vi "一体站流程自动启动.vi"(11 "参数":T1={"CODCr"={"启动测量模式"={"测量模式"=enum."水样测量"}, "确定按钮"=TRUE}, "参数启用"={"多参数"=FALSE, "CODMn"=FALSE, "总磷总氮"=FALSE, "氨氮"=FALSE, "CODcr"=FALSE}}) -> ()   [LabVIEW 2016, in "PLC.lvlib"]
uses:
  PLC.lvlib
  API/CodCr/CodCr.lvlib
panel:
  out "枚举":enum16{"初始化", "采配水启动", "等待", "配水", "排水", "结束"}(ring)
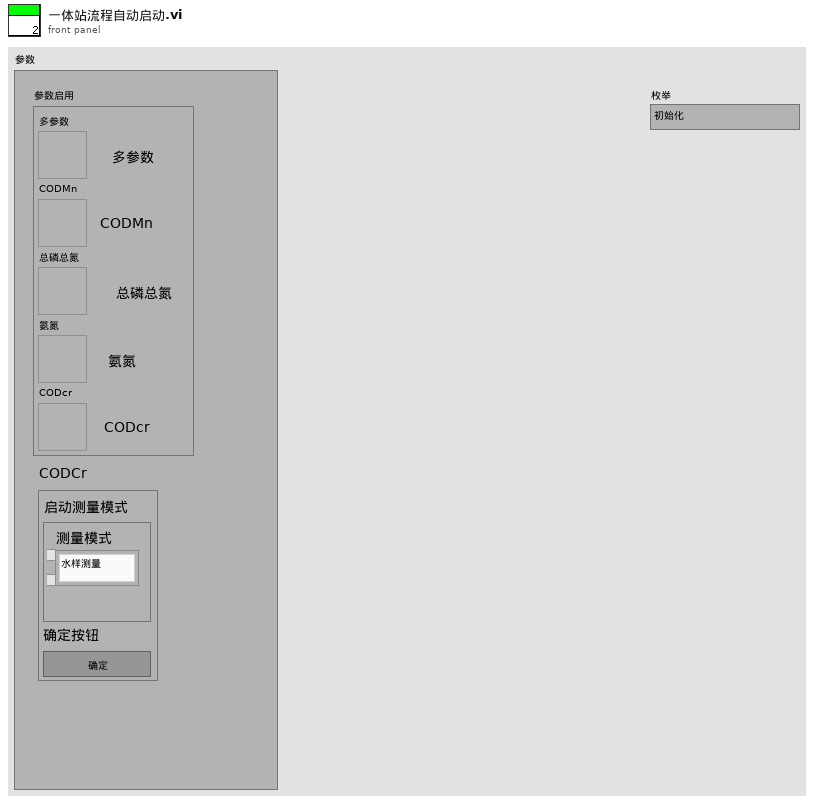
[diagram p1: front panel]
types:
  T1 = cluster{"CODCr":cluster{"启动测量模式":cluster{"测量模式":enum16{"水样测量", "标样核查", "零点核查", "跨度核查", "加标回收", "平行样", "校零", "校标"}}, "确定按钮":bool}, "参数启用":cluster{"多参数":bool, "CODMn":bool, "总磷总氮":bool, "氨氮":bool, "CODcr":bool}}
  T2 = cluster{"命令":string, cluster{"starting address":u16, "holding register value":u16}}
  T3 = cluster{"测量模式":enum16{"水样测量", "标样核查", "零点核查", "跨度核查", "空白测试", "加标回收", "平行样", "校零", "校标"}}
  T4 = cluster{"时间标识":timestamp, "设备":string, "日志信息":string, "流程参数":string}
  T5 = cluster{"时间标识":timestamp, "设备":string, "日志信息":string}
  T6 = enum16{"空闲", "水样测试", "标样核查", "零点核查", "跨度核查", "空白测试", "平行样测试", "加标回收", "空白校准", "标样校准", "初始化（清洗）"}
  T7 = enum16{"待机", "启动氨氮", "氨氮测量中", "启动总磷", "总磷测量中", "结束"}
  T8 = cluster{"站号":u16, "量程切换":enum32{"H", "L", "AUTO"}, "控制命令":enum16{"启动测量", "标样核查", "零点核查", "跨度核查", "空白测试", "平行样测试", "加标回收", "空白校准", "标样校准", "初始化（清洗）", "停止测试", "仪器重启", "校时", "模式设置", "测量间隔设置"}, "模式设置":enum16{"待机", "连续模式", "周期模式", "定点模式", "受控模式", "手动模式"}, "测量间隔":u16}
  T9 = cluster{"测量模式":enum16{"待机", "水样测试", "标样核查", "零点核查", "跨度核查", "空白测试", "平行样测试", "加标回收", "空白校准", "标样校准", "初始化（清洗）"}, "数据标记表":string, "测量时间":dbl}
  T10 = enum16{"待机", "水样测试", "标样核查", "零点核查", "跨度核查", "空白测试", "平行样测试", "加标回收", "空白校准", "标样校准", "初始化（清洗）"}
  T11 = cluster{"R0":i16, "R1":i16, "R2":i16, "R3":i16, "R4":i16, "R5":i16, "R6":i16, "R7":i16, "R8":i16, "R9":i16, "R10":i16, "R11":i16, "R12":i16, "R13":i16, "R14":i16, "R15":i16, "R16":i16, "R17":i16, "R18":i16, "R19":i16, "R20":i16, "R21":i16, "R22":i16, "R23":i16, "R24":i16, "R25":i16}
  T12 = enum32{"Bad", "Idle", "Run top level", "Running"}
  T13 = cluster{"系统时间":timestamp, "工作状态":enum16{"空闲", "水样测试", "标样核查", "零点核查", "跨度核查", "空白测试", "平行样测试", "加标回收", "空白校准", "标样校准", "初始化（清洗）"}, "测量模式":enum16{"待机", "连续模式", "周期模式", "定点模式", "受控模式", "手动模式"}, "告警代码":enum16{"无告警", "缺试剂告警", "缺水样告警", "缺蒸馏水告警", "缺标液告警", "仪表漏液告警", "标定异常告警", "超量程告警", "加热异常", "低试剂预警", "超上限告警", "超下限告警", "仪表内部其他异常", "滴定异常告警", "电极异常告警", "量程切换告警", "参数设置告警", "PH电极电位异常", "电导率电极异常", "浊度光度异常", "溶解氧电极异常", "溶解氧光强异常", "温度异常告警", "PH异常告警", "溶解氧异常告警", "电导率异常告警", "浊度异常告警", "叶绿素异常告警", "藻密度异常告警", "蓝绿藻异常告警", "ORP异常告警", "氨氮异常告警", "清洁刷异常告警", "SD卡异常告警", "蓝牙异常告警", "Wifi异常告警", "流程异常告警"}, "故障代码":enum16{"无故障", "电机故障", "温度故障", "通讯故障", "滴定故障"}, "日志代码":u16, "软件版本":u16, "F0":sgl, "F1":sgl, "F2":sgl, "F3":sgl, "T":sgl, "H":sgl, "id":u16, "flowid":u16, "量程":u16}
  T14 = cluster{"测量模式":enum16{"水样测量", "标样核查", "零点核查", "跨度核查", "加标回收", "平行样", "校零", "校标"}}
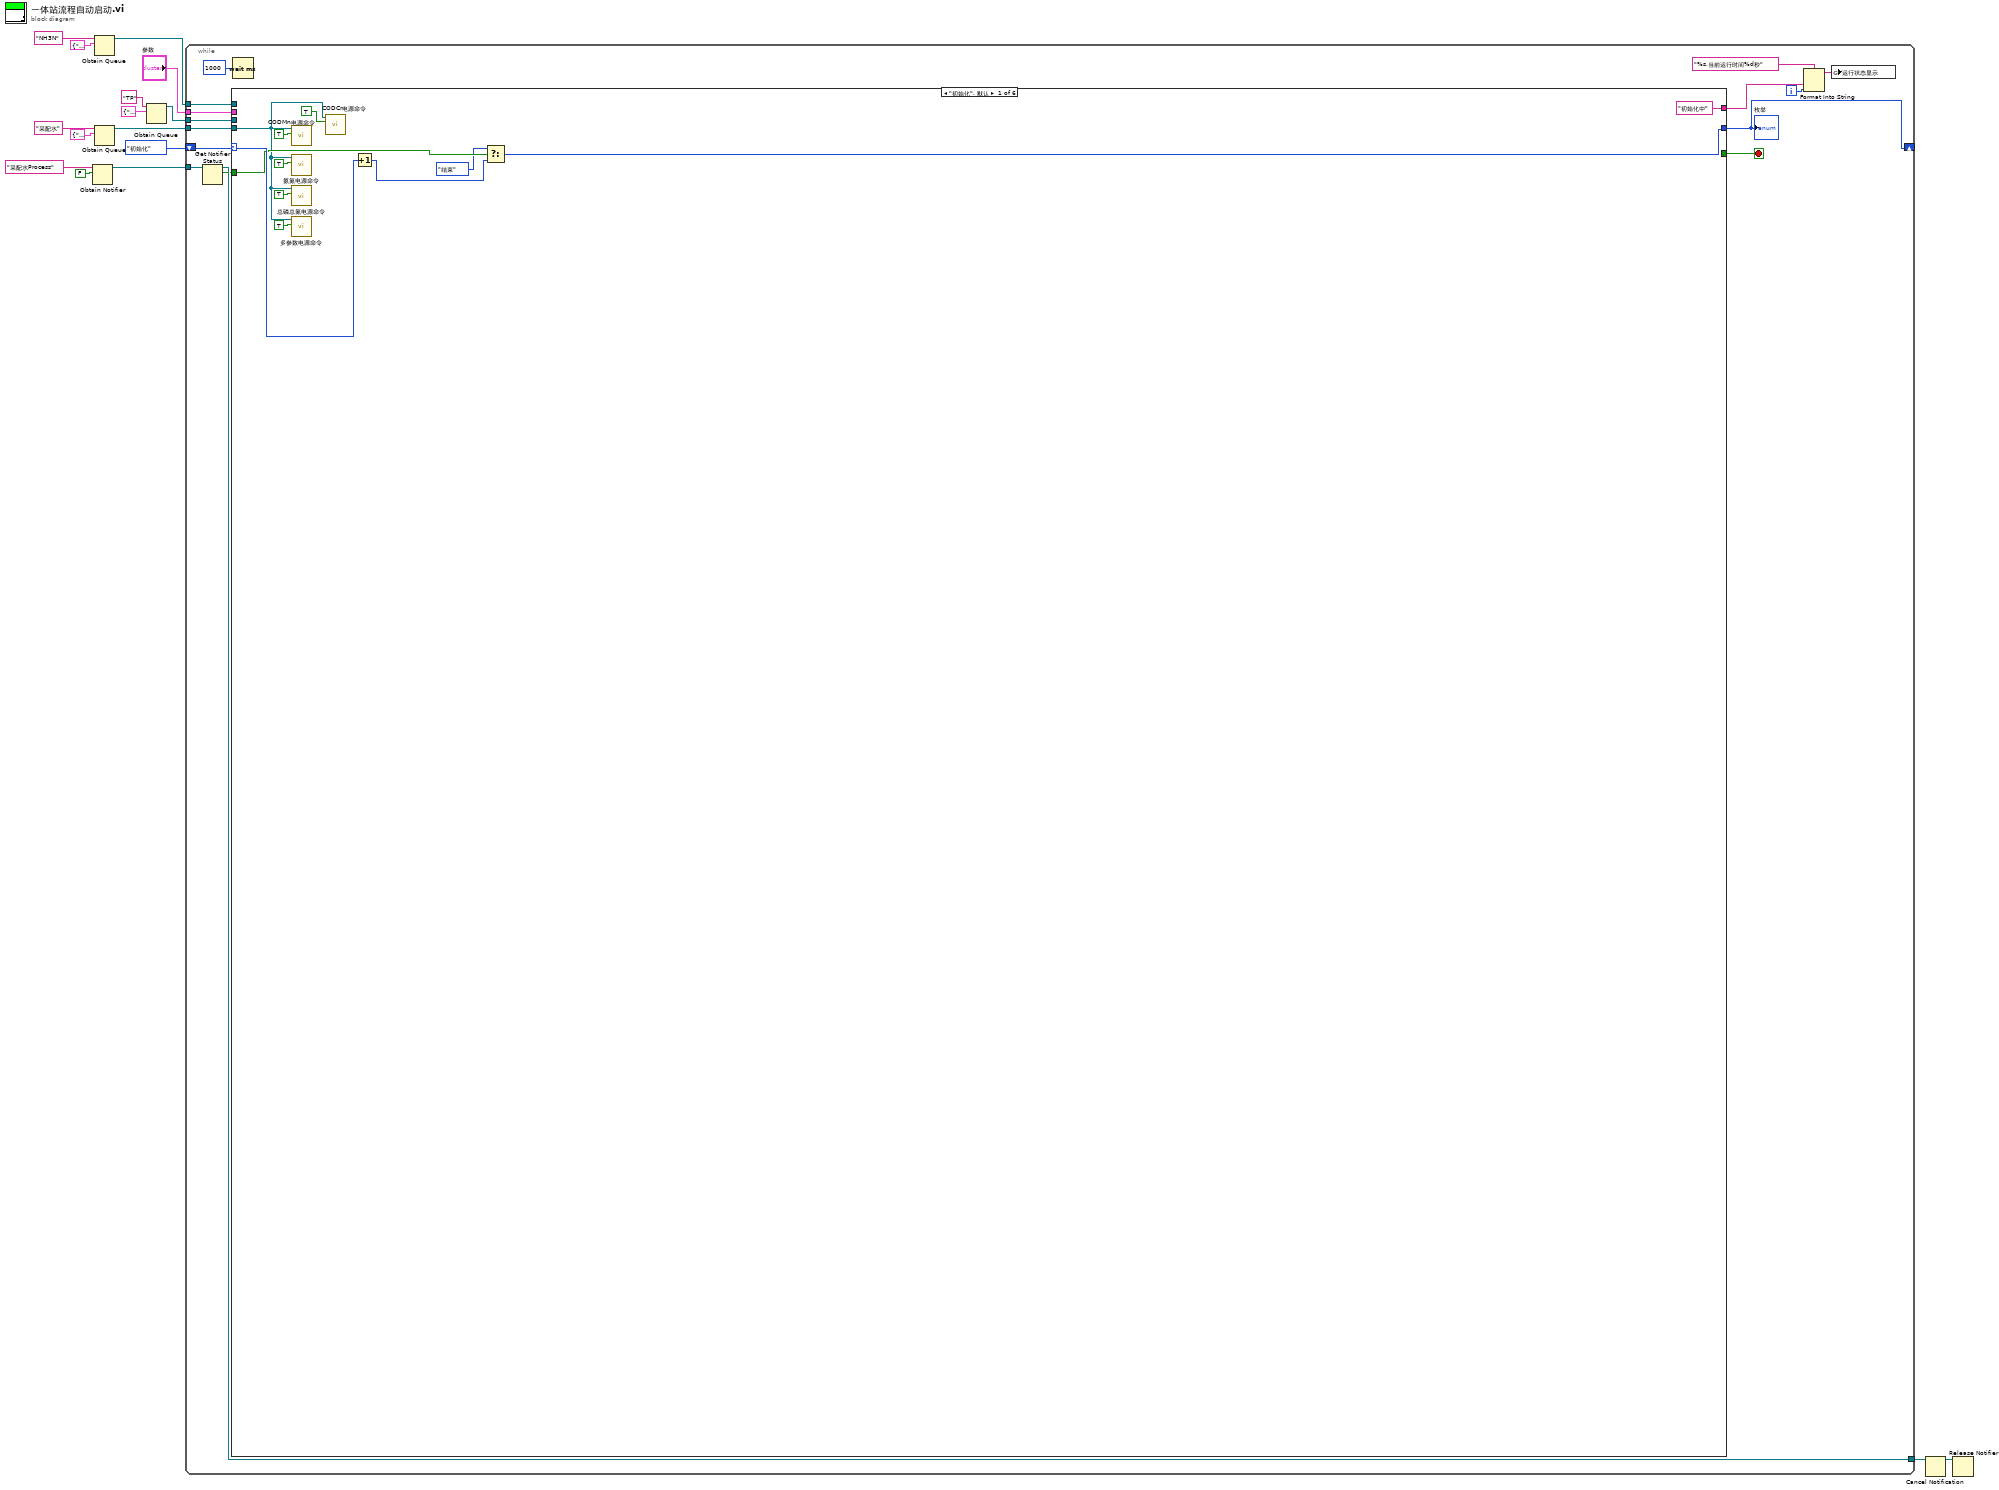
[diagram p0: block diagram]
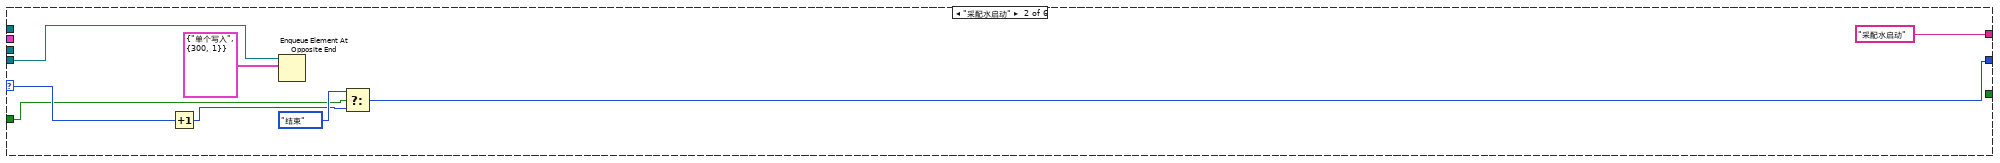
[diagram p2: hidden frame]
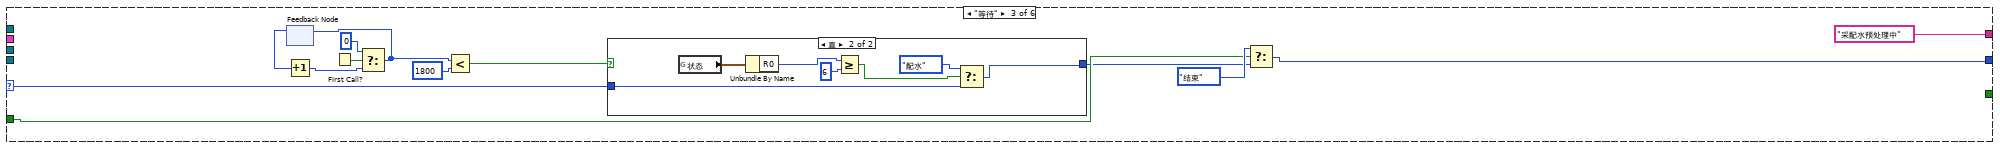
[diagram p3: hidden frame]
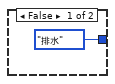
[diagram p4: hidden frame]
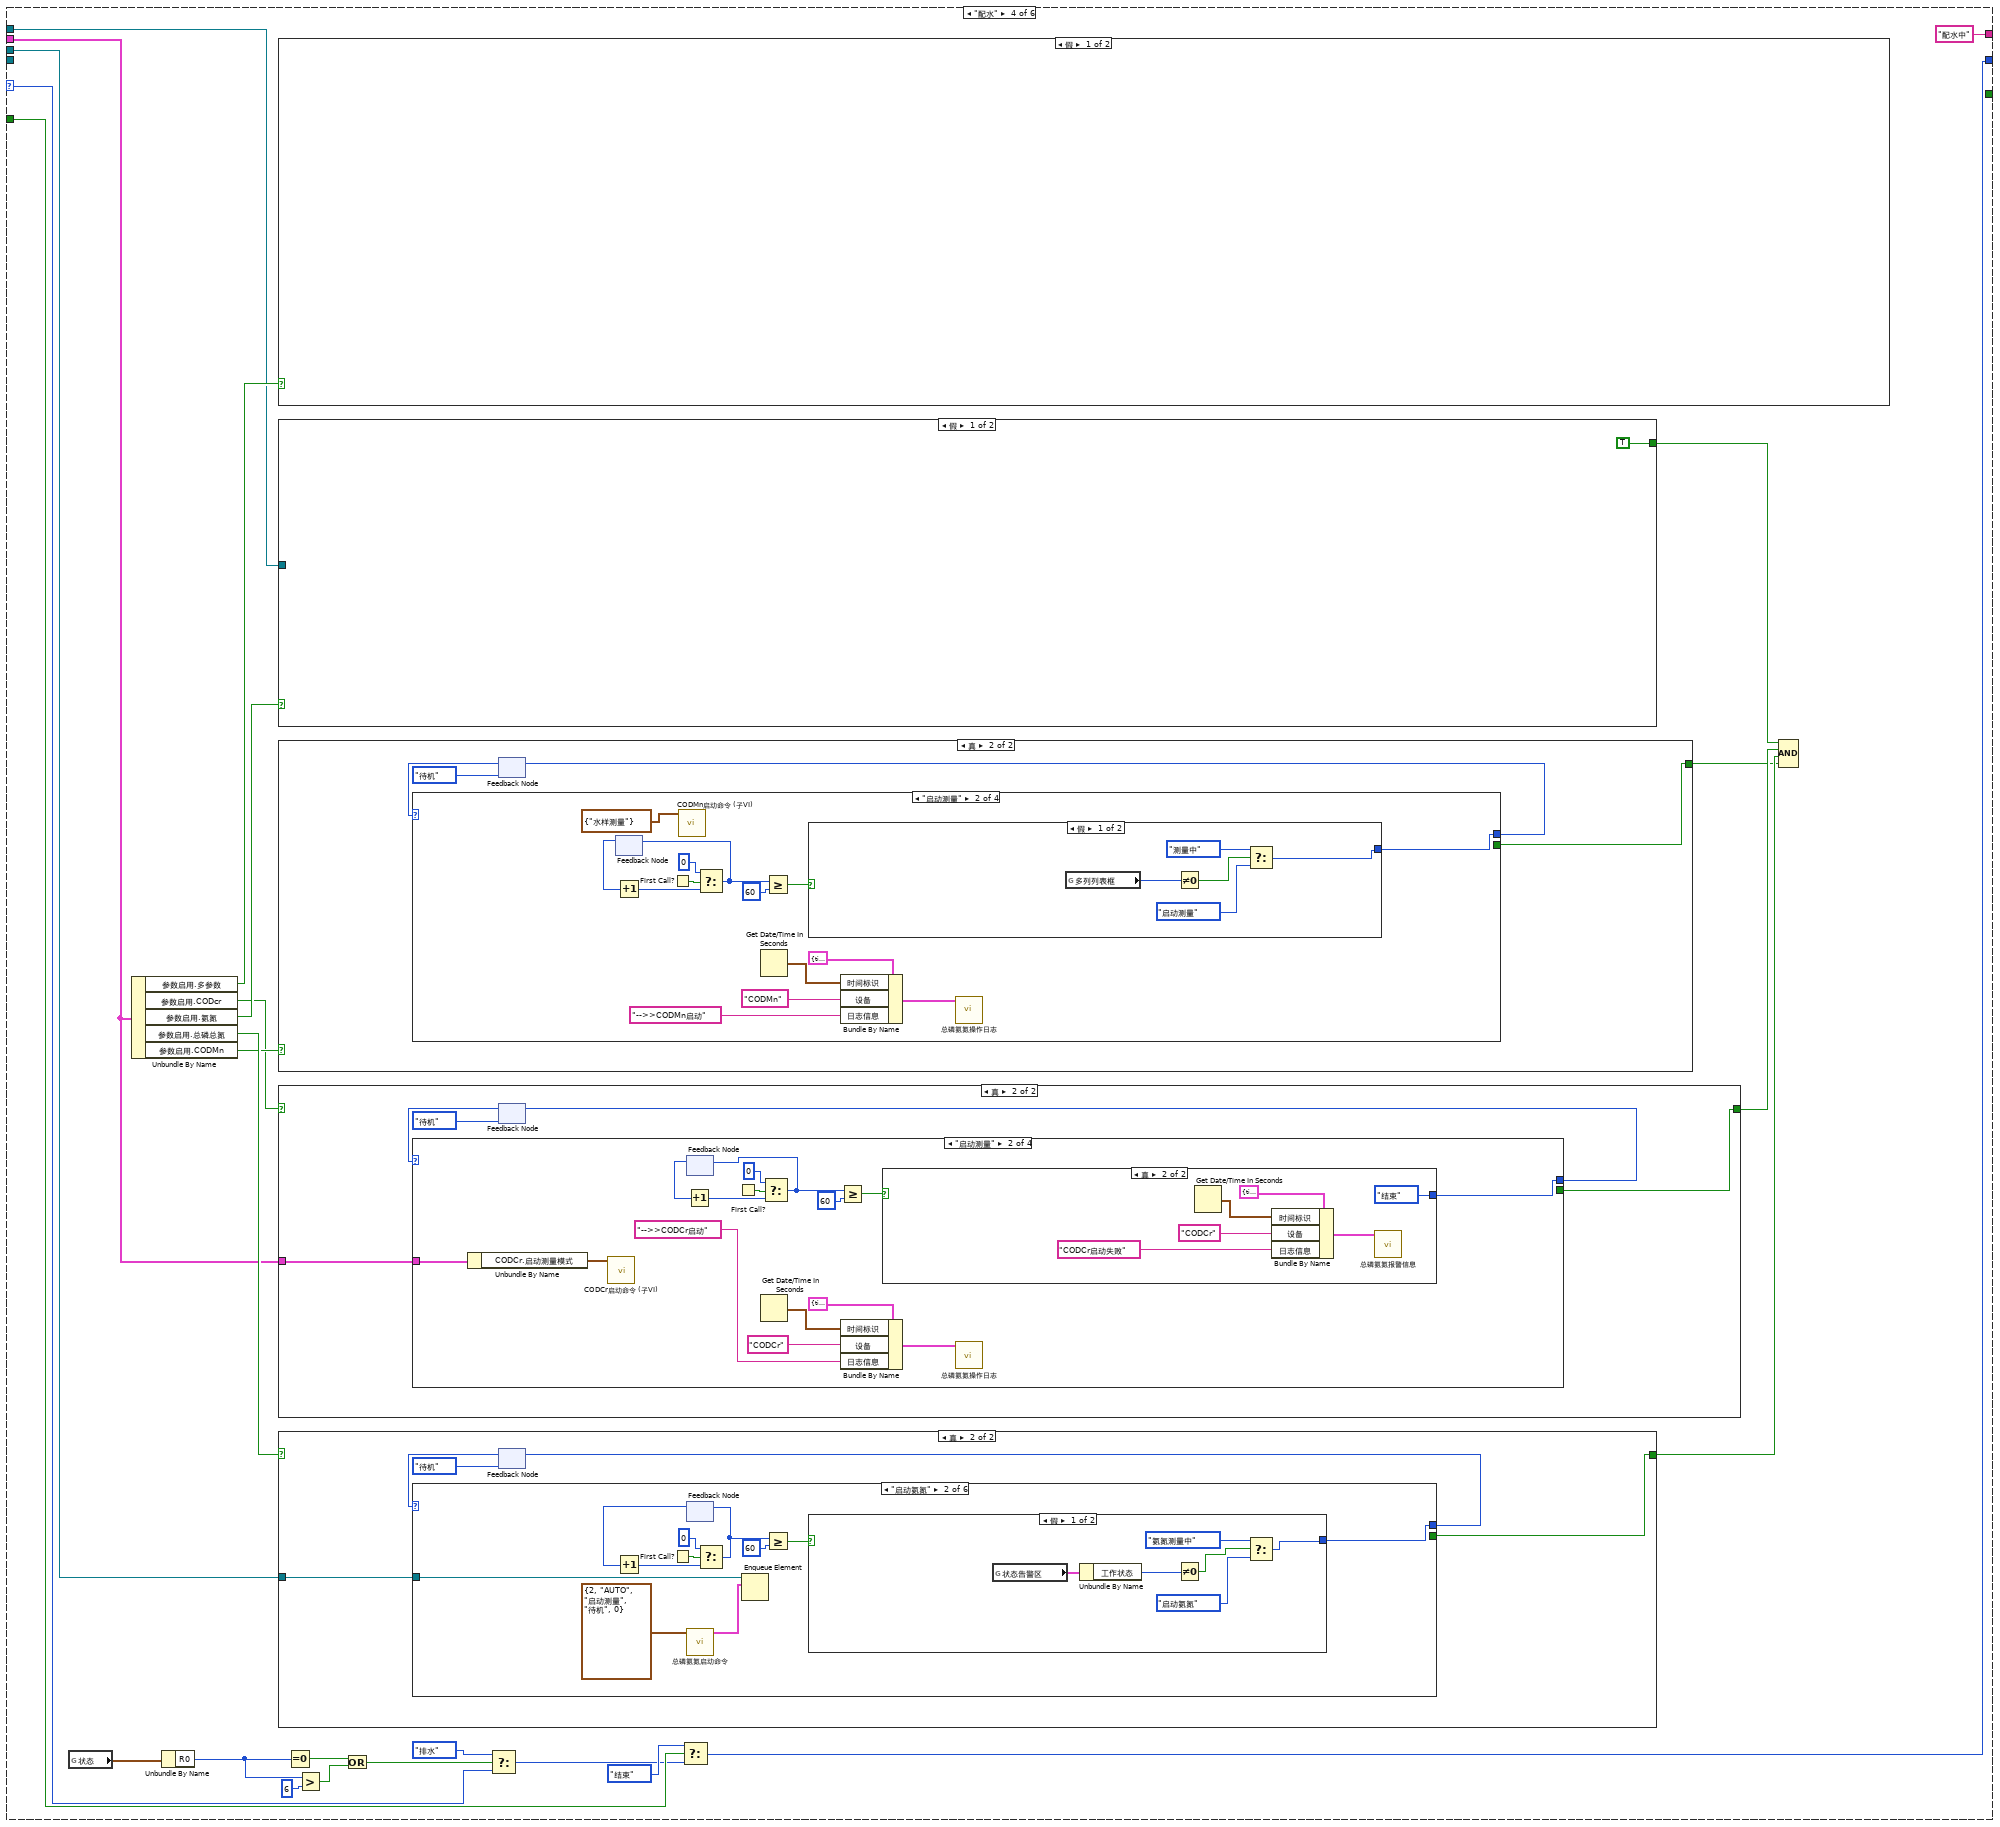
[diagram p5: hidden frame]
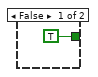
[diagram p6: hidden frame]
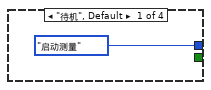
[diagram p7: hidden frame]
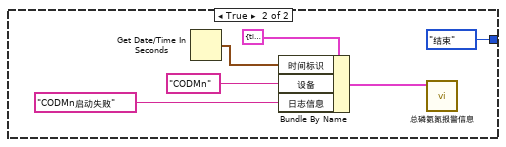
[diagram p8: hidden frame]
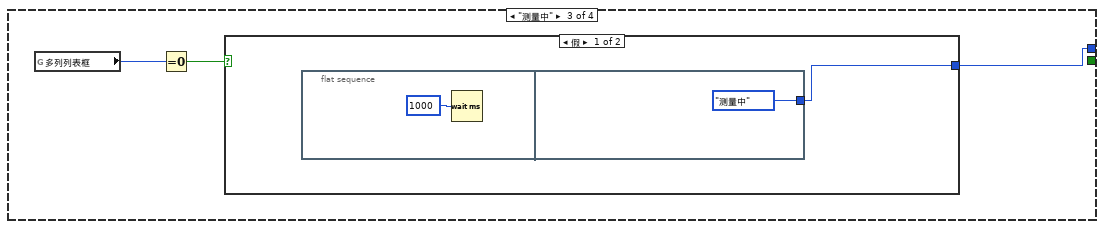
[diagram p9: hidden frame]
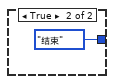
[diagram p10: hidden frame]
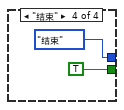
[diagram p11: hidden frame]
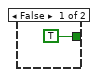
[diagram p12: hidden frame]
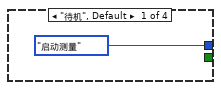
[diagram p13: hidden frame]
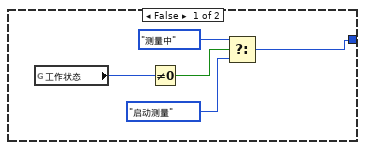
[diagram p14: hidden frame]
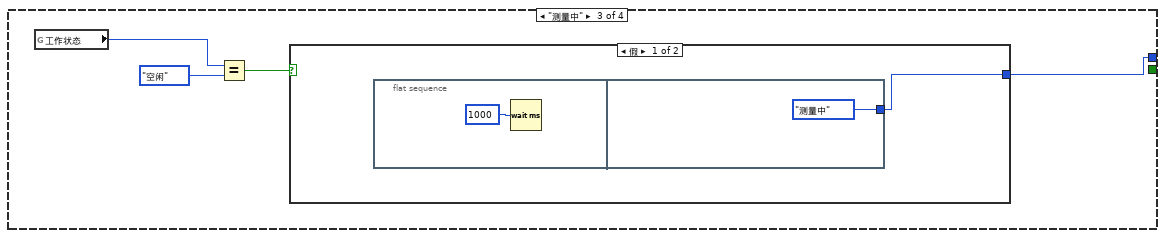
[diagram p15: hidden frame]
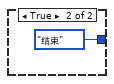
[diagram p16: hidden frame]
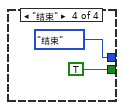
[diagram p17: hidden frame]
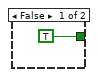
[diagram p18: hidden frame]
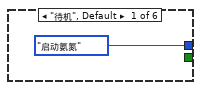
[diagram p19: hidden frame]
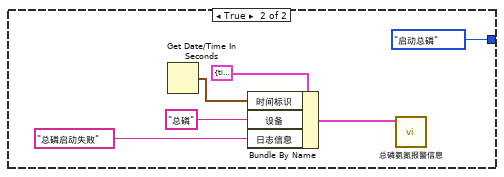
[diagram p20: hidden frame]
diagram:
  n1 = Obtain Notifier(name (unnamed)="采配水Process" ("名称（未命名）"), notification data type=FALSE) -> (notifier out=w7:refnum<notifier>)  [unwired: 2 in, 2 out]
  n2 = Obtain Queue(name (unnamed)="NH3N" ("名称（未命名）"), element data type=cluster{"命令":string, "data":variant} {"命令"="", "data"=variant}) -> (queue out=w2:refnum<queue>)  [unwired: 3 in, 2 out]
  n3 = Obtain Queue(name (unnamed)="采配水" ("名称（未命名）"), element data type=cluster{"命令":string, "数据":variant} {"命令"="", "数据"=variant}) -> (queue out=w14:refnum<queue>)  [unwired: 3 in, 2 out]
  n4 = Obtain Queue(name (unnamed)="TP" ("名称（未命名）"), element data type=cluster{"命令":string, "data":variant} {"命令"="", "data"=variant}) -> (queue out=w1:refnum<queue>)  [unwired: 3 in, 2 out]
  n5 = while {
    tunnel: w14 -> [w31]
    shift-right: [w29] -> _
    shift-left: enum16{"初始化", "采配水启动", "等待", "配水", "排水", "结束"}."初始化" ("枚举") -> [w30]
    tunnel: w2 -> [w27]
    tunnel: "参数" -> [w26]
    tunnel: w7 -> [w25]
    tunnel: [w24] -> w6
    tunnel: w1 -> [w18]
    i -> [w21]
    stop <- w20 stop-if-true
    n6 = Get Notifier Status(notifier=w25) -> (notifier out=w24:refnum<notifier>, current notification=w19:bool)  [unwired: 1 in, 3 out]
    n7 = case shown="\"初始化\", 默认" w30 {
      selector: w30 -> [w43 w49 w62 w96 w357 w363]
      tunnel: w31 -> [w33 w50 _ _ w358 _]
      tunnel: [w39 w44 w52 w91 w352 w362] -> w29
      tunnel: [_ _ _ _ _ TRUE] -> w20
      tunnel: w27 -> [_ _ _ w86 _ _]
      tunnel: w26 -> [_ _ _ w82 _ _]
      tunnel: ["初始化中" ("输入 1") "采配水启动" ("输入 1") "采配水预处理中" ("输入 1") "配水中" ("输入 1") "排水中" ("输入 1") "结束" ("输入 1")] -> w22
      tunnel: w19 -> [w41 w46 w54 w93 w354 _]
      tunnel: w18 -> [_ _ _ w87 _ _]
      frame "初始化", Default {
        n8 = call "CODMn电源命令.vi"("通电/断电"=TRUE, "队列"=w33) -> ()  [unwired: 9 in, 1 out]
        n9 = call "氨氮电源命令.vi"("通电/断电"=TRUE, "队列"=w33) -> ()  [unwired: 9 in, 1 out]
        n10 = call "总磷总氮电源命令.vi"("通电/断电"=TRUE, "队列"=w33) -> ()  [unwired: 9 in, 1 out]
        n11 = call "多参数电源命令.vi"("通电/断电"=TRUE, "队列"=w33) -> ()  [unwired: 9 in, 1 out]
        n12 = call "CODCr电源命令.vi"("通电/断电"=TRUE, "队列"=w33) -> ()  [unwired: 9 in, 1 out]
        n13 = Increment(x=w43) -> (x+1=w40:enum16{"初始化", "采配水启动", "等待", "配水", "排水", "结束"})
        n14 = Select(t=enum16{"初始化", "采配水启动", "等待", "配水", "排水", "结束"}."结束", s=w41, f=w40) -> (s? t:f=w39:enum16{"初始化", "采配水启动", "等待", "配水", "排水", "结束"})
      }
      frame "采配水启动" {
        n15 = Increment(x=w49) -> (x+1=w45:enum16{"初始化", "采配水启动", "等待", "配水", "排水", "结束"})
        n16 = Enqueue Element At Opposite End(queue=w50, element=T2 {"命令"="单个写入", {"starting address"=300, "holding register value"=1}} ("元素")) -> ()  [unwired: 2 in, 3 out]
        n17 = Select(t=enum16{"初始化", "采配水启动", "等待", "配水", "排水", "结束"}."结束", s=w46, f=w45) -> (s? t:f=w44:enum16{"初始化", "采配水启动", "等待", "配水", "排水", "结束"})
      }
      frame "等待" {
        n18 = feedback #1() -> (w59:i32)  [unwired: 1 in]
        n19 = Increment(x=w59) -> (x+1=w58:i32)
        n20 = First Call?() -> (First Call?: T/F=w60:bool)
        n21 = Select(t=0, s=w60, f=w58) -> (s? t:f=w57:i32)
        n22 = feedback-in #1(w57) -> ()
        n23 = Less?(x=w57, y=1800) -> (x < y?=w63:bool)
        n24 = case shown="真" w63 {
          tunnel: w62 -> [_ w67]
          tunnel: [enum16{"初始化", "采配水启动", "等待", "配水", "排水", "结束"}."排水" ("枚举") w66] -> w53
          frame False {
          }
          frame True {
            n25 = global read "采配水全局变量.vi" "状态"() -> (w72:T11)
            n26 = Unbundle By Name(w72) -> ("R0"=w71:i16)
            n27 = Greater Or Equal?(x=w71, y=i16 6) -> (x >= y?=w69:bool)
            n28 = Select(t=enum16{"初始化", "采配水启动", "等待", "配水", "排水", "结束"}."配水" ("枚举"), s=w69, f=w67) -> (s? t:f=w66:enum16{"初始化", "采配水启动", "等待", "配水", "排水", "结束"})
          }
        }
        n29 = Select(t=enum16{"初始化", "采配水启动", "等待", "配水", "排水", "结束"}."结束", s=w54, f=w53) -> (s? t:f=w52:enum16{"初始化", "采配水启动", "等待", "配水", "排水", "结束"})
      }
      frame "配水" {
        n30 = global read "采配水全局变量.vi" "状态"() -> (w78:T11)
        n31 = Unbundle By Name(w82) -> ("参数启用.多参数"=w90:bool, "参数启用.CODcr"=w81:bool, "参数启用.氨氮"=w89:bool, "参数启用.总磷总氮"=w88:bool, "参数启用.CODMn"=w83:bool)
        n32 = Unbundle By Name(w78) -> ("R0"=w77:i16)
        n33 = case shown="假" w90 {
          frame False {
          }
          frame True {
            n34 = feedback #2(enum16{"init", "启动仪器", "测量中"}."init") -> (w329:enum16{"init", "启动仪器", "测量中"})
            n35 = case shown="\"启动仪器\"" w329 {
              selector: w329 -> [w332 w337 _]
              tunnel: [w331 w336 enum16{"init", "启动仪器", "测量中"}."测量中"] -> w330
              frame "init", Default {
                n36 = Increment(x=w332) -> (x+1=w331:enum16{"init", "启动仪器", "测量中"})
              }
              frame "启动仪器" {
                n37 = vi-ref "斯坦道仪器.lvlib:五参数水样测试.vi"() -> (w334:refnum<vi>)
                n38 = property class="VI"(reference=w334) -> ("Name"=w333:string, "Exec.State"=w335:T12)  [unwired: 1 in, 2 out]
                n39 = case shown="\"Idle\"" w335 {
                  tunnel: w333 -> [_ w344]
                  frame "Bad", Default {
                  }
                  frame "Idle" {
                    n40 = global read "系统变量.vi" "运行模式"() -> (w339:enum16{"维护模式", "常规模式", "应急模式", "质控模式"})
                    n41 = case shown="\"常规模式\", 默认" w339 {
                      tunnel: ["M" ("数据标记表") "N" ("数据标记表")] -> w338
                      frame "维护模式" {
                      }
                      frame "常规模式", Default {
                      }
                    }
                    n42 = Bundle By Name(cluster=T9 {"测量模式"=enum."待机", "数据标记表"="", "测量时间"=0.0} ("启动参数"), "测量模式"=T10."水样测试", "数据标记表"=w338, "测量时间"=10.0) -> (w340:T9)
                    n43 = Open VI Reference(type specifier VI Refnum (for type only)=refnum<vi> refnum ("类型说明符VI引用句柄（仅用于类型）"), vi path=w344, options=128 ("选项")) -> (vi reference=w343:refnum<vi>)  [unwired: 3 in, 1 out]
                    n44 = call-by-ref "开始异步调用"(reference=w343, "启动参数"=w340) -> (reference out=w342:refnum<vi>)  [unwired: 12 in, 1 out]
                    n45 = Close Reference(reference=w342) -> ()  [unwired: 1 in, 1 out]
                  }
                }
                n46 = Increment(x=w337) -> (x+1=w336:enum16{"init", "启动仪器", "测量中"})
              }
              frame "测量中" {
              }
            }
            n47 = feedback-in #2(w330) -> ()
          }
        }
        n48 = case shown="假" w89 {
          tunnel: [TRUE w257] -> w85
          tunnel: w86 -> [_ w256]
          frame False {
          }
          frame True {
            n49 = feedback #3(T7."待机") -> (w259:T7)
            n50 = case shown="\"启动总磷\"" w259 {
              tunnel: [T7."启动氨氮" w272 w286 w304 w318 T7."结束"] -> w258
              tunnel: [_ _ _ _ _ TRUE] -> w257
              tunnel: w256 -> [_ w263 _ w295 _ _]
              frame "待机", Default {
              }
              frame "启动氨氮" {
                n51 = First Call?() -> (First Call?: T/F=w270:bool)
                n52 = feedback #4() -> (w269:i32)  [unwired: 1 in]
                n53 = Increment(x=w269) -> (x+1=w268:i32)
                n54 = call "总磷氨氮启动命令.vi"("参数"=T8 {"站号"=3, "量程切换"=enum."AUTO", "控制命令"=enum."启动测量", "模式设置"=enum."待机", "测量间隔"=0}) -> ("启动命令"=w264:cluster{"命令":string, "data":variant})  [unwired: 10 in]
                n55 = Select(t=0, s=w270, f=w268) -> (s? t:f=w267:i32)
                n56 = feedback-in #4(w267) -> ()
                n57 = Enqueue Element(queue=w263, element=w264) -> ()  [unwired: 2 in, 3 out]
                n58 = Greater Or Equal?(x=w267, y=60) -> (x >= y?=w265:bool)
                n59 = case shown="假" w265 {
                  tunnel: [w276 T7."结束"] -> w272
                  frame False {
                    n60 = global read "VAR总磷氨氮全局变量.vi" "状态告警区"() -> (w273:T13)
                    n61 = Unbundle By Name(w273) -> ("工作状态"=w278:T6)
                    n62 = Not Equal To 0?(x=w278) -> (x != 0?=w277:bool)
                    n63 = Select(t=T7."氨氮测量中", s=w277, f=T7."启动氨氮") -> (s? t:f=w276:T7)
                  }
                  frame True {
                    n64 = Get Date/Time In Seconds() -> (seconds since 1Jan1904=w283:timestamp)
                    n65 = Bundle By Name(cluster=T5 {"时间标识"=timestamp(0 s since 1904-01-01), "设备"="", "日志信息"=""} ("data in"), "时间标识"=w283, "设备"="氨氮", "日志信息"="氨氮启动失败") -> (w279:T5)
                    n66 = call "总磷氨氮报警信息.vi"("data in"=w279) -> ()  [unwired: 11 in]
                  }
                }
              }
              frame "氨氮测量中" {
                n67 = global read "VAR总磷氨氮全局变量.vi" "状态告警区"() -> (w285:T13)
                n68 = Unbundle By Name(w285) -> ("工作状态"=w288:T6, "id"=w287:u16)
                n69 = case shown="\"水样测试\", 默认" w288 {
                  tunnel: [T7."结束" w290] -> w286
                  tunnel: w287 -> [_ w291]
                  frame "空闲" {
                  }
                  frame "水样测试", Default {
                    n70 = case shown="76, 默认" w291 {
                      tunnel: [T7."氨氮测量中" T7."总磷测量中"] -> w290
                      frame 76, Default {
                      }
                      frame 131 {
                      }
                    }
                  }
                }
              }
              frame "启动总磷" {
                n71 = First Call?() -> (First Call?: T/F=w302:bool)
                n72 = call "总磷氨氮启动命令.vi"("参数"=T8 {"站号"=1, "量程切换"=enum."AUTO", "控制命令"=enum."启动测量", "模式设置"=enum."待机", "测量间隔"=0}) -> ("启动命令"=w296:cluster{"命令":string, "data":variant})  [unwired: 10 in]
                n73 = feedback #5() -> (w301:i32)  [unwired: 1 in]
                n74 = Increment(x=w301) -> (x+1=w300:i32)
                n75 = Select(t=0, s=w302, f=w300) -> (s? t:f=w299:i32)
                n76 = feedback-in #5(w299) -> ()
                n77 = Enqueue Element(queue=w295, element=w296) -> ()  [unwired: 2 in, 3 out]
                n78 = Greater Or Equal?(x=w299, y=60) -> (x >= y?=w297:bool)
                n79 = case shown="假" w297 {
                  tunnel: [w308 T7."结束"] -> w304
                  frame False {
                    n80 = global read "VAR总磷氨氮全局变量.vi" "状态告警区"() -> (w305:T13)
                    n81 = Unbundle By Name(w305) -> ("工作状态"=w309:T6)
                    n82 = Not Equal To 0?(x=w309) -> (x != 0?=w310:bool)
                    n83 = Select(t=T7."总磷测量中", s=w310, f=T7."启动总磷") -> (s? t:f=w308:T7)
                  }
                  frame True {
                    n84 = Get Date/Time In Seconds() -> (seconds since 1Jan1904=w316:timestamp)
                    n85 = Bundle By Name(cluster=T5 {"时间标识"=timestamp(0 s since 1904-01-01), "设备"="", "日志信息"=""} ("data in"), "时间标识"=w316, "设备"="总磷", "日志信息"="总磷启动失败") -> (w311:T5)
                    n86 = call "总磷氨氮报警信息.vi"("data in"=w311) -> ()  [unwired: 11 in]
                  }
                }
              }
              frame "总磷测量中" {
                n87 = global read "VAR总磷氨氮全局变量.vi" "状态告警区"() -> (w317:T13)
                n88 = Unbundle By Name(w317) -> ("工作状态"=w320:T6, "id"=w319:u16)
                n89 = case shown="\"水样测试\", 默认" w320 {
                  tunnel: [T7."结束" w322] -> w318
                  tunnel: w319 -> [_ w323]
                  frame "空闲" {
                  }
                  frame "水样测试", Default {
                    n90 = case shown="76, 默认" w323 {
                      tunnel: [T7."氨氮测量中" T7."总磷测量中"] -> w322
                      frame 76, Default {
                      }
                      frame 131 {
                      }
                    }
                  }
                }
              }
              frame "结束" {
              }
            }
            n91 = feedback-in #3(w258) -> ()
          }
        }
        n92 = case shown="真" w83 {
          tunnel: [TRUE w99] -> w79
          frame False {
          }
          frame True {
            n93 = feedback #6(enum16{"待机", "启动测量", "测量中", "结束"}."待机") -> (w101:enum16{"待机", "启动测量", "测量中", "结束"})
            n94 = case shown="\"启动测量\"" w101 {
              tunnel: [enum16{"待机", "启动测量", "测量中", "结束"}."启动测量" w117 w131 enum16{"待机", "启动测量", "测量中", "结束"}."结束"] -> w100
              tunnel: [_ _ _ TRUE] -> w99
              frame "待机", Default {
              }
              frame "启动测量" {
                n95 = feedback #7() -> (w113:i32)  [unwired: 1 in]
                n96 = Increment(x=w113) -> (x+1=w114:i32)
                n97 = First Call?() -> (First Call?: T/F=w112:bool)
                n98 = call "CODMn启动命令 (子VI).vi"("启动测量模式"=T3 {"测量模式"=enum."水样测量"}) -> ()  [unwired: 11 in]
                n99 = Select(t=0, s=w112, f=w114) -> (s? t:f=w115:i32)
                n100 = feedback-in #7(w115) -> ()
                n101 = Get Date/Time In Seconds() -> (seconds since 1Jan1904=w109:timestamp)
                n102 = Greater Or Equal?(x=w115, y=60) -> (x >= y?=w110:bool)
                n103 = case shown="假" w110 {
                  tunnel: [w119 enum16{"待机", "启动测量", "测量中", "结束"}."结束"] -> w117
                  frame False {
                    n104 = global read "运行时序全局变量.vi" "多列列表框"() -> (w118:i32)
                    n105 = Not Equal To 0?(x=w118) -> (x != 0?=w120:bool)
                    n106 = Select(t=enum16{"待机", "启动测量", "测量中", "结束"}."测量中", s=w120, f=enum16{"待机", "启动测量", "测量中", "结束"}."启动测量") -> (s? t:f=w119:enum16{"待机", "启动测量", "测量中", "结束"})
                  }
                  frame True {
                    n107 = Get Date/Time In Seconds() -> (seconds since 1Jan1904=w123:timestamp)
                    n108 = Bundle By Name(cluster=T5 {"时间标识"=timestamp(0 s since 1904-01-01), "设备"="", "日志信息"=""} ("data in"), "时间标识"=w123, "设备"="CODMn", "日志信息"="CODMn启动失败") -> (w127:T5)
                    n109 = call "总磷氨氮报警信息.vi"("data in"=w127) -> ()  [unwired: 11 in]
                  }
                }
                n110 = Bundle By Name(cluster=T4 {"时间标识"=timestamp(0 s since 1904-01-01), "设备"="", "日志信息"="", "流程参数"=""} ("data in"), "时间标识"=w109, "设备"="CODMn", "日志信息"="-->>CODMn启动") -> (w105:T4)
                n111 = call "总磷氨氮操作日志.vi"("data in"=w105) -> ()  [unwired: 11 in]
              }
              frame "测量中" {
                n112 = global read "运行时序全局变量.vi" "多列列表框"() -> (w130:i32)
                n113 = Equal To 0?(x=w130) -> (x = 0?=w129:bool)
                n114 = case shown="假" w129 {
                  tunnel: [w132 enum16{"待机", "启动测量", "测量中", "结束"}."结束"] -> w131
                  frame False {
                    n115 = flat-sequence {
                      tunnel: [enum16{"待机", "启动测量", "测量中", "结束"}."测量中"] -> w132
                      frame #0 {
                        n116 = Wait (ms)(milliseconds to wait=u32 1000 ("等待时间（毫秒）")) -> ()  [unwired: 1 out]
                      }
                      frame #1 {
                      }
                    }
                  }
                  frame True {
                  }
                }
              }
              frame "结束" {
              }
            }
            n117 = feedback-in #6(w100) -> ()
          }
        }
        n118 = case shown="真" w81 {
          tunnel: [TRUE w140] -> w80
          tunnel: w82 -> [_ w139]
          frame False {
          }
          frame True {
            n119 = feedback #8(enum16{"待机", "启动测量", "测量中", "结束"}."待机") -> (w142:enum16{"待机", "启动测量", "测量中", "结束"})
            n120 = case shown="\"启动测量\"" w142 {
              tunnel: [enum16{"待机", "启动测量", "测量中", "结束"}."启动测量" w158 w174 enum16{"待机", "启动测量", "测量中", "结束"}."结束"] -> w141
              tunnel: w139 -> [_ w159 _ _]
              tunnel: [_ _ _ TRUE] -> w140
              frame "待机", Default {
              }
              frame "启动测量" {
                n121 = Unbundle By Name(w159) -> ("CODCr.启动测量模式"=w157:T14)
                n122 = call "CODCr启动命令 (子VI).vi"("启动测量模式"=w157) -> ()  [unwired: 11 in]
                n123 = feedback #9() -> (w153:i32)  [unwired: 1 in]
                n124 = Increment(x=w153) -> (x+1=w154:i32)
                n125 = First Call?() -> (First Call?: T/F=w152:bool)
                n126 = Get Date/Time In Seconds() -> (seconds since 1Jan1904=w149:timestamp)
                n127 = Select(t=0, s=w152, f=w154) -> (s? t:f=w155:i32)
                n128 = feedback-in #9(w155) -> ()
                n129 = Greater Or Equal?(x=w155, y=60) -> (x >= y?=w150:bool)
                n130 = Bundle By Name(cluster=T4 {"时间标识"=timestamp(0 s since 1904-01-01), "设备"="", "日志信息"="", "流程参数"=""} ("data in"), "时间标识"=w149, "设备"="CODCr", "日志信息"="-->>CODCr启动") -> (w145:T4)
                n131 = case shown="真" w150 {
                  tunnel: [w160 enum16{"待机", "启动测量", "测量中", "结束"}."结束"] -> w158
                  frame False {
                    n132 = global read "CODCr工作状态.vi" "工作状态"() -> (w161:T6)
                    n133 = Not Equal To 0?(x=w161) -> (x != 0?=w162:bool)
                    n134 = Select(t=enum16{"待机", "启动测量", "测量中", "结束"}."测量中", s=w162, f=enum16{"待机", "启动测量", "测量中", "结束"}."启动测量") -> (s? t:f=w160:enum16{"待机", "启动测量", "测量中", "结束"})
                  }
                  frame True {
                    n135 = Get Date/Time In Seconds() -> (seconds since 1Jan1904=w165:timestamp)
                    n136 = Bundle By Name(cluster=T5 {"时间标识"=timestamp(0 s since 1904-01-01), "设备"="", "日志信息"=""} ("data in"), "时间标识"=w165, "设备"="CODCr", "日志信息"="CODCr启动失败") -> (w169:T5)
                    n137 = call "总磷氨氮报警信息.vi"("data in"=w169) -> ()  [unwired: 11 in]
                  }
                }
                n138 = call "总磷氨氮操作日志.vi"("data in"=w145) -> ()  [unwired: 11 in]
              }
              frame "测量中" {
                n139 = global read "CODCr工作状态.vi" "工作状态"() -> (w173:T6)
                n140 = Equal?(x=w173, y=T6."空闲" ("工作状态")) -> (x = y?=w172:bool)
                n141 = case shown="假" w172 {
                  tunnel: [w175 enum16{"待机", "启动测量", "测量中", "结束"}."结束"] -> w174
                  frame False {
                    n142 = flat-sequence {
                      tunnel: [enum16{"待机", "启动测量", "测量中", "结束"}."测量中"] -> w175
                      frame #0 {
                        n143 = Wait (ms)(milliseconds to wait=u32 1000 ("等待时间（毫秒）")) -> ()  [unwired: 1 out]
                      }
                      frame #1 {
                      }
                    }
                  }
                  frame True {
                  }
                }
              }
              frame "结束" {
              }
            }
            n144 = feedback-in #8(w141) -> ()
          }
        }
        n145 = case shown="真" w88 {
          tunnel: w87 -> [_ w183]
          tunnel: [TRUE w182] -> w84
          frame False {
          }
          frame True {
            n146 = feedback #10(T7."待机") -> (w185:T7)
            n147 = case shown="\"启动氨氮\"" w185 {
              tunnel: [T7."启动氨氮" w197 w211 w230 w244 T7."结束"] -> w184
              tunnel: w183 -> [_ w198 _ w231 _ _]
              tunnel: [_ _ _ _ _ TRUE] -> w182
              frame "待机", Default {
              }
              frame "启动氨氮" {
                n148 = First Call?() -> (First Call?: T/F=w195:bool)
                n149 = feedback #11() -> (w194:i32)  [unwired: 1 in]
                n150 = Increment(x=w194) -> (x+1=w193:i32)
                n151 = call "总磷氨氮启动命令.vi"("参数"=T8 {"站号"=2, "量程切换"=enum."AUTO", "控制命令"=enum."启动测量", "模式设置"=enum."待机", "测量间隔"=0}) -> ("启动命令"=w188:cluster{"命令":string, "data":variant})  [unwired: 10 in]
                n152 = Select(t=0, s=w195, f=w193) -> (s? t:f=w192:i32)
                n153 = feedback-in #11(w192) -> ()
                n154 = Enqueue Element(queue=w198, element=w188) -> ()  [unwired: 2 in, 3 out]
                n155 = Greater Or Equal?(x=w192, y=60) -> (x >= y?=w190:bool)
                n156 = case shown="假" w190 {
                  tunnel: [w201 T7."启动总磷"] -> w197
                  frame False {
                    n157 = global read "VAR总磷氨氮全局变量.vi" "状态告警区"() -> (w204:T13)
                    n158 = Unbundle By Name(w204) -> ("工作状态"=w203:T6)
                    n159 = Not Equal To 0?(x=w203) -> (x != 0?=w202:bool)
                    n160 = Select(t=T7."氨氮测量中", s=w202, f=T7."启动氨氮") -> (s? t:f=w201:T7)
                  }
                  frame True {
                    n161 = Get Date/Time In Seconds() -> (seconds since 1Jan1904=w209:timestamp)
                    n162 = Bundle By Name(cluster=T5 {"时间标识"=timestamp(0 s since 1904-01-01), "设备"="", "日志信息"=""} ("data in"), "时间标识"=w209, "设备"="总磷", "日志信息"="总磷启动失败") -> (w205:T5)
                    n163 = call "总磷氨氮报警信息.vi"("data in"=w205) -> ()  [unwired: 11 in]
                  }
                }
              }
              frame "氨氮测量中" {
                n164 = global read "VAR总磷氨氮全局变量.vi" "状态告警区"() -> (w214:T13)
                n165 = Unbundle By Name(w214) -> ("工作状态"=w213:T6, "id"=w212:u16)
                n166 = case shown="\"空闲\"" w213 {
                  tunnel: [T7."启动总磷" w217] -> w211
                  tunnel: w212 -> [_ w218]
                  frame "空闲" {
                    n167 = Wait (ms)(milliseconds to wait=u32 5000 ("等待时间（毫秒）")) -> ()  [unwired: 1 out]
                  }
                  frame "水样测试", Default {
                    n168 = case shown="131" w218 {
                      tunnel: [T7."氨氮测量中" T7."总磷测量中"] -> w217
                      frame 76, Default {
                      }
                      frame 131 {
                      }
                    }
                  }
                }
              }
              frame "启动总磷" {
                n169 = First Call?() -> (First Call?: T/F=w228:bool)
                n170 = feedback #12() -> (w227:i32)  [unwired: 1 in]
                n171 = Increment(x=w227) -> (x+1=w226:i32)
                n172 = call "总磷氨氮启动命令.vi"("参数"=T8 {"站号"=1, "量程切换"=enum."AUTO", "控制命令"=enum."启动测量", "模式设置"=enum."待机", "测量间隔"=0}) -> ("启动命令"=w221:cluster{"命令":string, "data":variant})  [unwired: 10 in]
                n173 = Select(t=0, s=w228, f=w226) -> (s? t:f=w225:i32)
                n174 = feedback-in #12(w225) -> ()
                n175 = Enqueue Element(queue=w231, element=w221) -> ()  [unwired: 2 in, 3 out]
                n176 = Greater Or Equal?(x=w225, y=60) -> (x >= y?=w223:bool)
                n177 = case shown="假" w223 {
                  tunnel: [w234 T7."结束"] -> w230
                  frame False {
                    n178 = global read "VAR总磷氨氮全局变量.vi" "状态告警区"() -> (w235:T13)
                    n179 = Unbundle By Name(w235) -> ("工作状态"=w236:T6)
                    n180 = Not Equal To 0?(x=w236) -> (x != 0?=w237:bool)
                    n181 = Select(t=T7."总磷测量中", s=w237, f=T7."启动总磷") -> (s? t:f=w234:T7)
                  }
                  frame True {
                    n182 = Get Date/Time In Seconds() -> (seconds since 1Jan1904=w243:timestamp)
                    n183 = Bundle By Name(cluster=T5 {"时间标识"=timestamp(0 s since 1904-01-01), "设备"="", "日志信息"=""} ("data in"), "时间标识"=w243, "设备"="总氮", "日志信息"="总氮启动失败") -> (w238:T5)
                    n184 = call "总磷氨氮报警信息.vi"("data in"=w238) -> ()  [unwired: 11 in]
                  }
                }
              }
              frame "总磷测量中" {
                n185 = global read "VAR总磷氨氮全局变量.vi" "状态告警区"() -> (w247:T13)
                n186 = Unbundle By Name(w247) -> ("工作状态"=w246:T6, "id"=w245:u16)
                n187 = case shown="\"空闲\"" w246 {
                  tunnel: [T7."结束" w249] -> w244
                  tunnel: w245 -> [_ w250]
                  frame "空闲" {
                  }
                  frame "水样测试", Default {
                    n188 = case shown="131" w250 {
                      tunnel: [T7."氨氮测量中" T7."总磷测量中"] -> w249
                      frame 76, Default {
                      }
                      frame 131 {
                      }
                    }
                  }
                }
              }
              frame "结束" {
              }
            }
            n189 = feedback-in #10(w184) -> ()
          }
        }
        n190 = Equal To 0?(x=w77) -> (x = 0?=w74:bool)
        n191 = Greater?(x=w77, y=i16 6) -> (0:w75:bool)
        n192 = Or(x=w74, y=w75) -> (x .or. y?=w73:bool)
        n193 = Select(t=enum16{"初始化", "采配水启动", "等待", "配水", "排水", "结束"}."排水" ("枚举"), s=w73, f=w96) -> (s? t:f=w92:enum16{"初始化", "采配水启动", "等待", "配水", "排水", "结束"})
        n194 = Select(t=enum16{"初始化", "采配水启动", "等待", "配水", "排水", "结束"}."结束", s=w93, f=w92) -> (s? t:f=w91:enum16{"初始化", "采配水启动", "等待", "配水", "排水", "结束"})
        n195 = Compound Arithmetic op=AND ("复合运算")(w85, w80, w84, w79) -> ()  [unwired: 1 out]
      }
      frame "排水" {
        n196 = Increment(x=w357) -> (x+1=w353:enum16{"初始化", "采配水启动", "等待", "配水", "排水", "结束"})
        n197 = Enqueue Element At Opposite End(queue=w358, element=T2 {"命令"="单个写入", {"starting address"=303, "holding register value"=1}} ("元素")) -> ()  [unwired: 2 in, 3 out]
        n198 = Select(t=enum16{"初始化", "采配水启动", "等待", "配水", "排水", "结束"}."结束", s=w354, f=w353) -> (s? t:f=w352:enum16{"初始化", "采配水启动", "等待", "配水", "排水", "结束"})
      }
      frame "结束" {
        n199 = Increment(x=w363) -> (x+1=w362:enum16{"初始化", "采配水启动", "等待", "配水", "排水", "结束"})
      }
    }
    "枚举" <- w29
    n200 = Wait (ms)(milliseconds to wait=u32 1000 ("等待时间（毫秒）")) -> ()  [unwired: 1 out]
    n201 = Format Into String(format string="%s,当前运行时间%d秒" ("格式字符串"), w22, w21) -> (resulting string=w17:string)  [unwired: 2 in, 1 out]
    n202 = global write "采配水全局变量.vi" "运行状态显示"(w17) -> ()
  }
  n203 = Cancel Notification(0:w6) -> (8:w5:refnum<notifier>)  [unwired: 1 in, 2 out]
  n204 = Release Notifier(notifier=w5) -> ()  [unwired: 2 in, 3 out]
